vi "fpga_W&R_ADC_W_DACs_Write_then_CLK.vi"() -> ()   [LabVIEW 2018]
uses:
  <vilib>/rvi/Emulation/niFpgaGetClockAttributes.vi
  <vilib>/rvi/Emulation/niFpgaSctlEmulationGetInTimedLoop.vi
  <vilib>/rvi/Emulation/niFpgaEmulationReportErrorSimple.vi
  <vilib>/rvi/eio/common/nirviEmuTemplateMethod_errors.vi
  <vilib>/rvi/Emulation/niFpgaCriticalErrorInLSC.vi
  <vilib>/eio/EIONode/EIONode.xnode
panel:
  in  "DAC 3 write":bool[](array[boolean])=[FALSE, FALSE, FALSE, FALSE, FALSE, FALSE, FALSE, FALSE, FALSE, FALSE, FALSE, FALSE, FALSE, FALSE, FALSE, FALSE]
  in  "DAC 2 write":bool[](array[boolean])=[FALSE, FALSE, FALSE, FALSE, FALSE, FALSE, FALSE, FALSE, FALSE, FALSE, FALSE, FALSE, FALSE, FALSE, FALSE, FALSE]
  in  "DAC 1 write":bool[](array[boolean])=[FALSE, FALSE, FALSE, FALSE, FALSE, FALSE, FALSE, FALSE, FALSE, FALSE, FALSE, FALSE, FALSE, FALSE, FALSE, FALSE]
  out "ADC read":bool[](array[boolean])
  in  "ADC write":bool[](array[boolean])=[FALSE, FALSE, FALSE, FALSE, FALSE, TRUE, FALSE, FALSE, FALSE, FALSE, FALSE, FALSE, FALSE, FALSE, FALSE, FALSE]
  in  "delay (ticks)":u32=800
  in  "Stop":bool
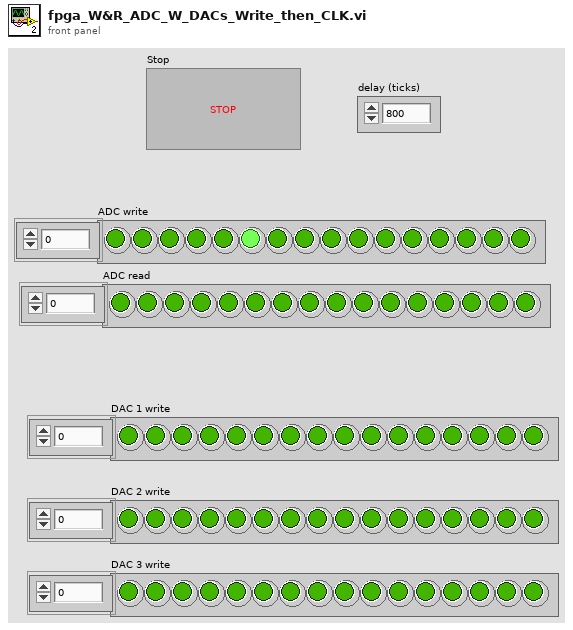
[diagram p1: front panel]
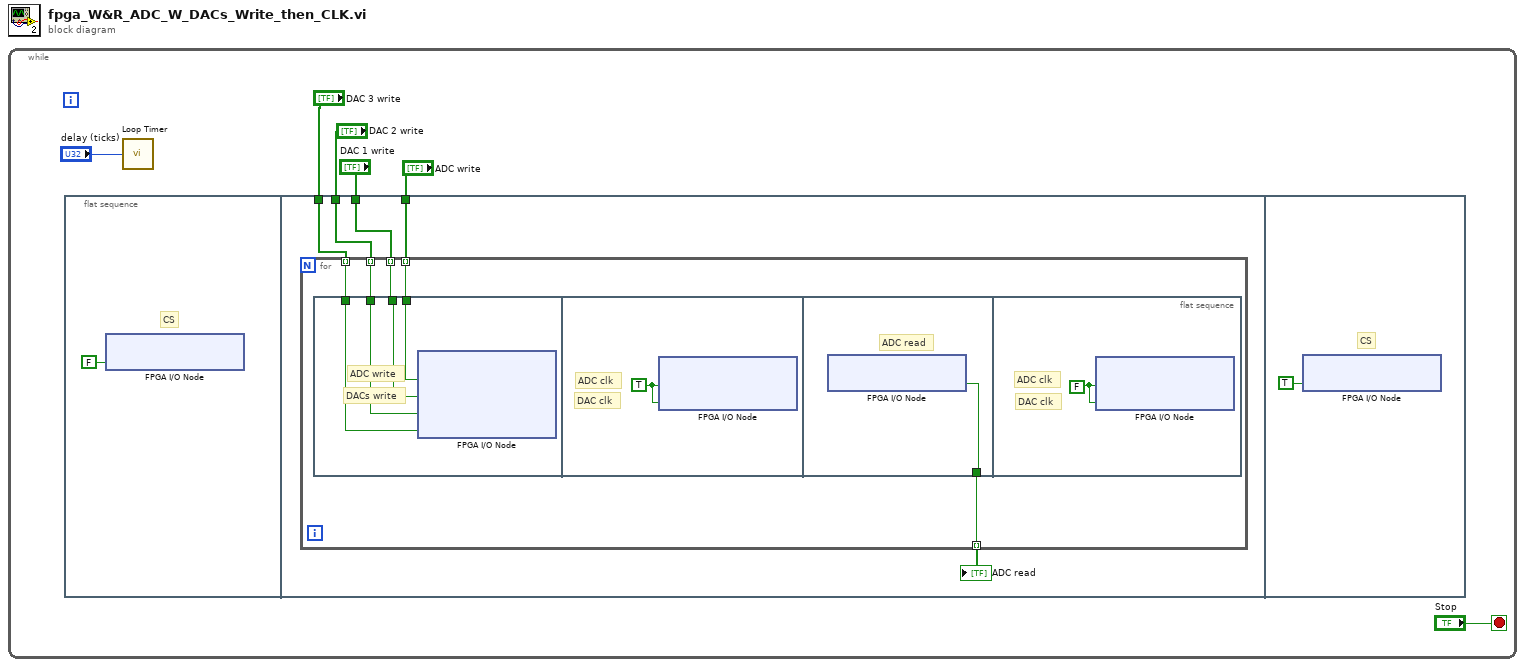
[diagram p0: block diagram]
diagram:
  n1 = while {
    stop <- "Stop" stop-if-true
    n2 = flat-sequence {
      tunnel: "ADC write" -> [w12]
      tunnel: "DAC 1 write" -> [w10]
      tunnel: "DAC 2 write" -> [w9]
      tunnel: "DAC 3 write" -> [w8]
      frame #0 {
        # "CS"
        n3 = xnode "FPGA I/O Node"("ConnectorA/DIO4"=FALSE) -> ()  [unwired: 1 in, 1 out]
      }
      frame #1 {
        n4 = for {
          tunnel: w12 -> [w17] mode=indexing
          tunnel: [w16] -> w11 mode=indexing
          tunnel: w10 -> [w15] mode=indexing
          tunnel: w9 -> [w14] mode=indexing
          tunnel: w8 -> [w13] mode=indexing
          n5 = flat-sequence {
            tunnel: w17 -> [w21]
            tunnel: w15 -> [w20]
            tunnel: w14 -> [w19]
            tunnel: w13 -> [w18]
            tunnel: [w23] -> w16
            frame #0 {
              # "DACs write"
              # "ADC write"
              n6 = xnode "FPGA I/O Node"("ConnectorA/DIO2"=w21, "ConnectorA/DIO6"=w20, "ConnectorA/DIO7"=w19, "ConnectorA/DIO8"=w18) -> ()  [unwired: 4 in, 4 out]
            }
            frame #1 {
              w22 = TRUE ("ConnectorA/DIO3")
              # "DAC clk"
              # "ADC clk"
              n7 = xnode "FPGA I/O Node"("ConnectorA/DIO3"=w22, "ConnectorA/DIO5"=w22) -> ()  [unwired: 2 in, 2 out]
            }
            frame #2 {
              # "ADC read"
              n8 = xnode "FPGA I/O Node"() -> ("ConnectorA/DIO1"=w23:bool)  [unwired: 1 in, 1 out]
            }
            frame #3 {
              w24 = FALSE ("ConnectorA/DIO3")
              # "DAC clk"
              # "ADC clk"
              n9 = xnode "FPGA I/O Node"("ConnectorA/DIO3"=w24, "ConnectorA/DIO5"=w24) -> ()  [unwired: 2 in, 2 out]
            }
          }
        }
        "ADC read" <- w11
      }
      frame #2 {
        # "CS"
        n10 = xnode "FPGA I/O Node"("ConnectorA/DIO4"=TRUE) -> ()  [unwired: 1 in, 1 out]
      }
    }
    n11 = call "Loop Timer"("Count(Ticks)"="delay (ticks)") -> ()  [unwired: 1 out]
  }
